vi "Get Server Operation.vi"(8 "error in (no error)":errorcluster, 11 "Server Message in":refnum<class "Server Message.lvclass">) -> (0 "error out":errorcluster, 2 "Server Operation":T1, 3 "Server Message out":refnum<class "Server Message.lvclass">)   [LabVIEW 2022 SP3, in "obs-websocket-lv.lvlib" / "Server Message.lvclass"]
uses:
  Server Message.lvclass
  Server Message.lvclass/Server Message.ctl
  Server Operation.ctl
  obs-websocket-lv.lvlib
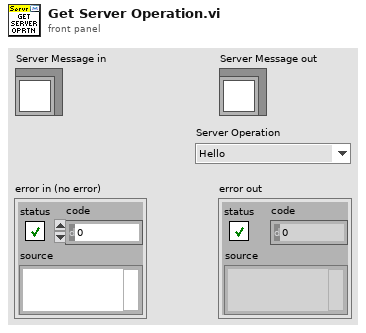
[diagram p1: front panel]
types:
  T1 = typedef "obs-websocket-lv.lvlib/Server Operation.ctl" = enum16{"Hello", "Identified", "Event", "RequestResponse", "RequestBatchResponse"}
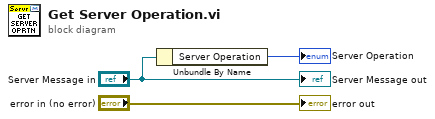
[diagram p0: block diagram]
diagram:
  n1 = Unbundle By Name("Server Message in") -> ("Server Operation"=→"Server Operation":T1)
  "error out" <- "error in (no error)"
  "Server Message out" <- "Server Message in"
